vi "Analyse.vi"(8 "error in (no error)":errorcluster, 10 "Image in":T1, 11 "Coin Analyser in":refnum<class "Coin Analyser.lvclass">) -> (0 "error out":errorcluster, 1 "Coins":cluster{"x":i32, "y":i32, "diameter":i32}[](array[cluster]), 2 "Image Out":T1, 3 "Coin Analyser out":refnum<class "Coin Analyser.lvclass">)   [LabVIEW 2022 SP3, in "Coin Analyser.lvclass"]
uses:
  Coin Analyser.lvclass
  <vilib>/vision/Image Controls.llb/IMAQ Image.ctl
  Coins.ctl
  Coin Analyser.lvclass/Coin Analyser.ctl
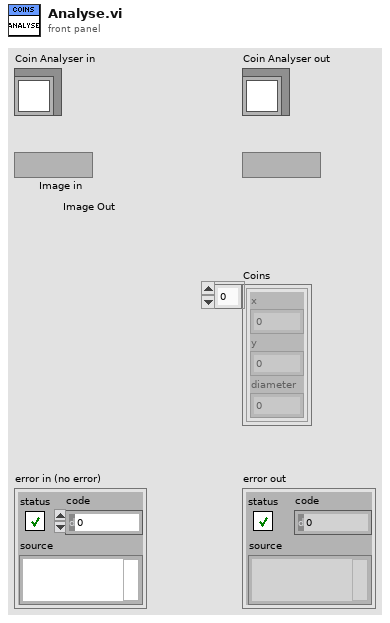
[diagram p1: front panel]
types:
  T1 = typedef "IMAQ Image.ctl" = refnum<image>
  T2 = typedef "Coin Analyser.lvclass/Coins.ctl" = cluster{"x":i32, "y":i32, "diameter":i32}
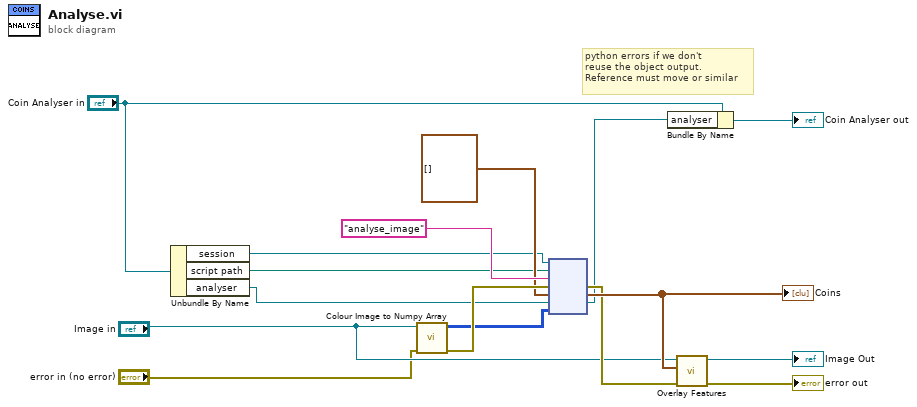
[diagram p0: block diagram]
diagram:
  # "python errors if we don't\nreuse the object output.\nReference must move or similar"
  n1 = Unbundle By Name("Coin Analyser in") -> ("session"=w4:refnum<k35>, "script path"=w6:path, "analyser"=w5:refnum<k38>)
  n2 = call "Colour Image to Numpy Array.vi"("error in (no error)"="error in (no error)", "Refnum in"="Image in") -> ("error out"=w15:errorcluster, "Array"=w12:u8[][][])  [unwired: 8 in]
  n3 = node(w4, w6, "analyse_image" ("function name"), w15, T2[] [], w5, w12) -> (w11:errorcluster, w13:T2[], w2:refnum<k38>)  [unwired: 1 in, 3 out]
  "Coins" <- w13
  n4 = Bundle By Name(cluster="Coin Analyser in", "analyser"=w2) -> (→"Coin Analyser out":refnum<class "Coin Analyser.lvclass">)
  n5 = call "Overlay Features.vi"("error in (no error)"=w11, "Features"=w13, "Refnum in"="Image in") -> ("Error Out"=→"error out":errorcluster, "Refnum out"=→"Image Out":T1)  [unwired: 7 in]
